vi "Draft.vi"() -> ()   [LabVIEW 2018]
uses:
  <vilib>/Utility/miscctls.llb/LVRowAndColumnUnsignedTypeDef.ctl
panel:
  in  "String":string="qweqweq"
  in  "Index Values":T1
  in  "Table Control":string[][](table)
  out "Boolean":bool
  in  "stop":bool
  in  "Numeric":u8
  out "Slide":u8(slide) scale=0.0..100.0
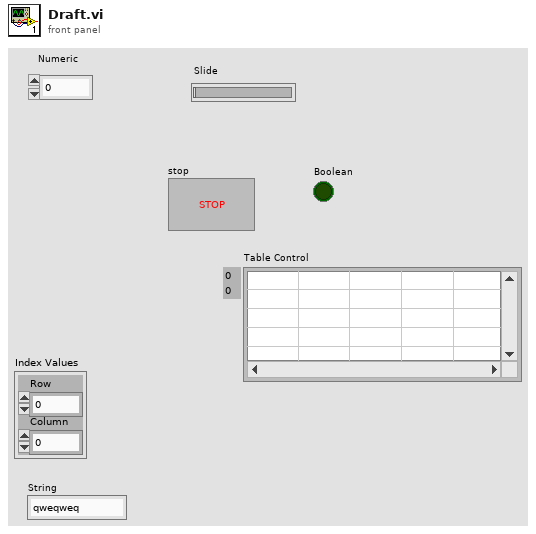
[diagram p1: front panel]
types:
  T1 = typedef "LVRowAndColumnUnsignedTypeDef.ctl" = cluster{"Row":u32, "Column":u32}
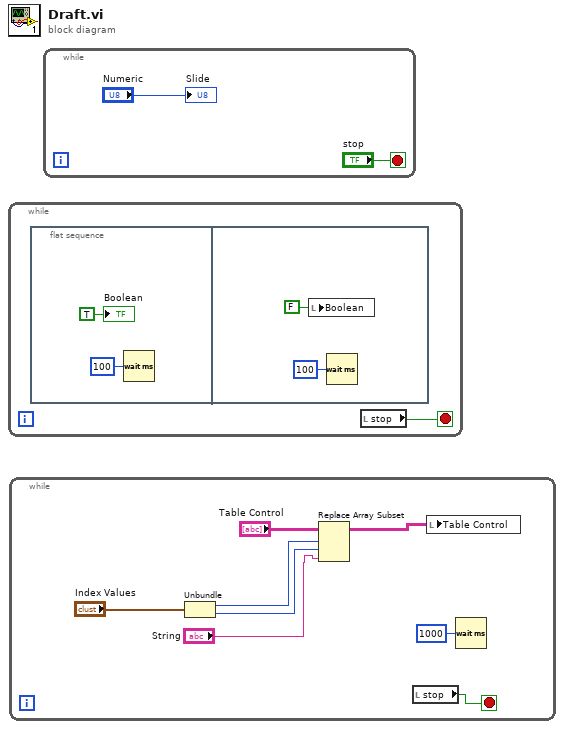
[diagram p0: block diagram]
diagram:
  n1 = while {
    stop <- w1 stop-if-true
    n2 = flat-sequence {
      frame #0 {
        n3 = Wait (ms)(milliseconds to wait=u32 100) -> ()  [unwired: 1 out]
        "Boolean" <- TRUE ("Boolean")
      }
      frame #1 {
        n4 = local write "Boolean"(FALSE ("Boolean")) -> ()
        n5 = Wait (ms)(milliseconds to wait=u32 100) -> ()  [unwired: 1 out]
      }
    }
    n6 = local read "stop"() -> (w1:bool)
  }
  n7 = while {
    stop <- w13 stop-if-true
    n8 = Unbundle("Index Values") -> ("Row"=w10:u32, "Column"=w9:u32)
    n9 = Replace Array Subset(array="Table Control", new element="String", index (row)=w10, index (col)=w9) -> (w8:string[][])
    n10 = local read "stop"() -> (w13:bool)
    n11 = local write "Table Control"(w8) -> ()
    n12 = Wait (ms)(milliseconds to wait=u32 1000) -> ()  [unwired: 1 out]
  }
  n13 = while {
    stop <- "stop" stop-if-true
    "Slide" <- "Numeric"
  }
